vi "fitting_side.vi"(9 "side of clusters":cluster{"Array out":dbl[][]}[](array[cluster]), 10 "ratio":dbl, 11 "side velocity threshold":dbl) -> (2 "D of clusters":cluster{"D":ext[]}[](array[cluster]), 3 "fitting clusters":cluster{"fitting array":dbl[][]}[](array[cluster]))   [LabVIEW 2017]
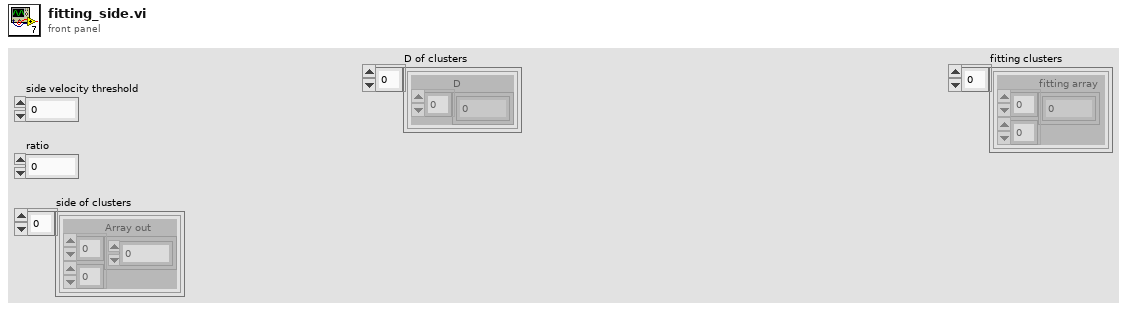
[diagram p1: front panel]
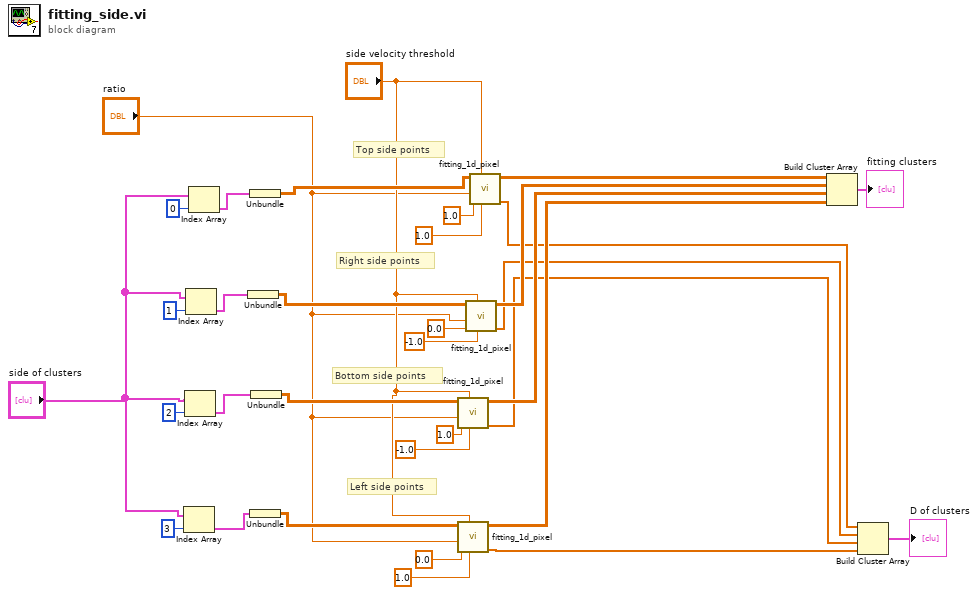
[diagram p0: block diagram]
diagram:
  # "Left side points"
  # "Bottom side points"
  # "Right side points"
  # "Top side points"
  n1 = Index Array(array="side of clusters", index=3 ("index (page)")) -> (element=w30:cluster{"Array out":dbl[][]})
  n2 = Index Array(array="side of clusters", index=2 ("index (page)")) -> (element=w29:cluster{"Array out":dbl[][]})
  n3 = Index Array(array="side of clusters", index=1 ("index (page)")) -> (element=w28:cluster{"Array out":dbl[][]})
  n4 = Index Array(array="side of clusters", index=0 ("index (page)")) -> (element=w26:cluster{"Array out":dbl[][]})
  n5 = Unbundle(w28) -> ("Array out"=w31:dbl[][])
  n6 = Unbundle(w26) -> ("Array out"=w27:dbl[][])
  n7 = Unbundle(w30) -> ("Array out"=w33:dbl[][])
  n8 = Unbundle(w29) -> ("Array out"=w32:dbl[][])
  n9 = call "fitting_1d_pixel.vi"("D sign"=-1.0, "side velocity threshold"="side velocity threshold", "fitting axis"=1.0, "ratio_pixel2mil"="ratio", "array in"=w32) -> ("D"=w3:ext[], "fitting array"=w8:dbl[][])  [unwired: 5 in]
  n10 = call "fitting_1d_pixel.vi"("D sign"=1.0, "side velocity threshold"="side velocity threshold", "fitting axis"=0.0, "ratio_pixel2mil"="ratio", "array in"=w33) -> ("D"=w2:ext[], "fitting array"=w7:dbl[][])  [unwired: 5 in]
  n11 = call "fitting_1d_pixel.vi"("D sign"=-1.0, "side velocity threshold"="side velocity threshold", "fitting axis"=0.0, "ratio_pixel2mil"="ratio", "array in"=w31) -> ("D"=w4:ext[], "fitting array"=w9:dbl[][])  [unwired: 5 in]
  n12 = call "fitting_1d_pixel.vi"("D sign"=1.0, "side velocity threshold"="side velocity threshold", "fitting axis"=1.0, "ratio_pixel2mil"="ratio", "array in"=w27) -> ("D"=w5:ext[], "fitting array"=w10:dbl[][])  [unwired: 5 in]
  n13 = Build Cluster Array(w10, w9, w8, w7) -> (→"fitting clusters":cluster{"fitting array":dbl[][]}[])
  n14 = Build Cluster Array(w5, w4, w3, w2) -> (→"D of clusters":cluster{"D":ext[]}[])
